vi "cfg serialize test.vi"() -> ()   [LabVIEW 2013, in "CVT Consuming Engine Tests.lvlib"]
uses:
  CVT Consuming Engine Tests.lvlib
  Configuration/CVT Engine Configuration.lvclass
panel:
  out "OK":bool
  out "error out":errorcluster
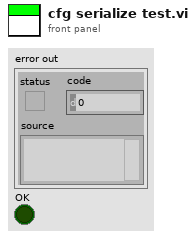
[diagram p1: front panel]
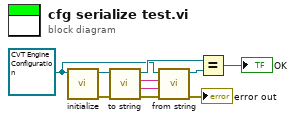
[diagram p0: block diagram]
diagram:
  w4 = refnum<class "CVT Engine Configuration.lvclass"> refnum ("CVT Engine Configuration")
  n1 = call-dynamic "initialize.vi"("configuration in"=w4) -> ("error out"=w9:errorcluster, "configuration out"=w10:refnum<class "CVT Engine Configuration.lvclass">)  [unwired: 8 in, 1 out]
  n2 = call-dynamic "to string.vi"("error in"=w9, "CVT Engine Configuration in"=w10) -> ("error out"=w8:errorcluster, "data"=w1:string, "version"=w2:string, "CVT Engine Configuration out"=w5:refnum<class "CVT Engine Configuration.lvclass">)  [unwired: 6 in]
  n3 = call-dynamic "from string.vi"("error in"=w8, "data"=w1, "version"=w2, "CVT Engine Configuration in"=w4) -> ("error out"=→"error out":errorcluster, "CVT Engine Configuration out"=w6:refnum<class "CVT Engine Configuration.lvclass">)  [unwired: 6 in]
  n4 = Equal?(x=w5, y=w6) -> (x = y?=→"OK":bool)
